vi "Initialize Buffer.vi"(4 "Error In":errorcluster) -> (0 "Error Out":errorcluster)   [LabVIEW 2015, in "Ramp Signal Data Buffer.lvlib"]
uses:
  Ramp Signal Data Buffer.lvlib
  _libraries/Startup Processes/_typedefs/Subpanel Names.ctl
  _libraries/Config Data/Config Data.lvclass
  _libraries/Startup Processes/Startup Processes.lvlib
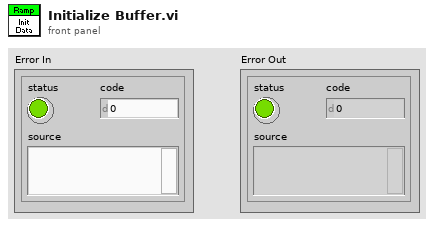
[diagram p1: front panel]
types:
  T1 = typedef "Startup Processes.lvlib/Subpanel Names.ctl" = enum16{"Sine Source", "Ramp Source", "Hen House TC", "Dog House TC", "Out House TC"}
  T2 = typedef "Ramp Signal Data Buffer.lvlib/buffer data typedef.ctl" = cluster{"Ramp Data":dbl[], "Counter":i32}
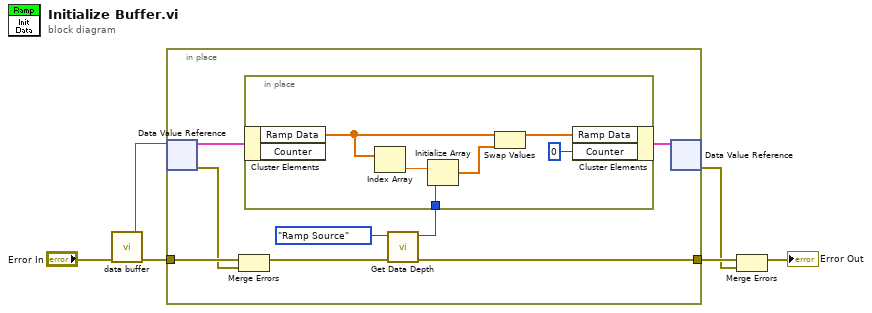
[diagram p0: block diagram]
diagram:
  n1 = call "data buffer.vi"("Error In"="Error In") -> ("Error Out"=w4:errorcluster, "DVR"=w5:refnum<data-value>)  [unwired: 5 in]
  n2 = in-place {
    in-place-border: w4 -> [w14]
    in-place-border: [w10] -> w3
    n3 = in-place-dvr #1(w5) -> (w9:T2, w13:errorcluster)
    n4 = Merge Errors(w14, w13) -> (w12:errorcluster)
    n5 = call "Get Data Depth.vi"("error in (no error)"=w12, "Depth to fetch"=Subpanel_Names."Ramp Source") -> ("error out"=w10:errorcluster, "Data Depth"=w11:i32)  [unwired: 4 in]
    n6 = in-place {
      in-place-border: w11 -> [w20]
      n7 = in-place-cluster #2(w9) -> ("Ramp Data"=w17:dbl[])  [unwired: 1 out]
      n8 = Index Array(array=w17) -> (element=w18:dbl)  [unwired: 1 in]
      n9 = Initialize Array(w18, w20) -> (w19:dbl[])
      n10 = Swap Values(12:w17, 14:w19) -> (1:w16:dbl[])  [unwired: 1 in, 1 out]
      n11 = in-place-cluster #2("Ramp Data"=w16, "Counter"=0) -> (w8:T2)
    }
    n12 = in-place-dvr #1(w8) -> (w1:errorcluster)  [unwired: 1 out]
  }
  n13 = Merge Errors(w3, w1) -> (→"Error Out":errorcluster)
